vi "PXI Atten to Multiplier.vi"(8 "error in (no error)":errorcluster, 11 "Attenuation":dbl) -> (0 "error out":errorcluster, 3 "Multiplier setting":dbl[](array[numeric])=[1.0, 0.001, 1.0, 1.0, 1.0, 1.0, 1.0, 1.0])   [LabVIEW 2020]
doc: "Set multiplier values by writing the config file.\nIt also changes the multiplier global variable."
uses:
  Utility VIs/Math VIs/dB to Linear (scalar).vi
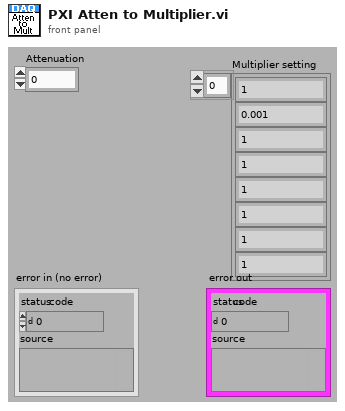
[diagram p1: front panel]
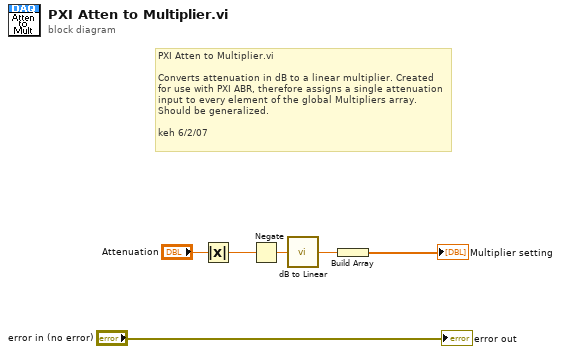
[diagram p0: block diagram]
diagram:
  # "PXI Atten to Multiplier.vi\n\nConverts attenuation in dB to a linear multiplier. Created for use with PXI ABR, therefore assigns a single attenuation input to every element of the global Multipliers array. Should be generalized.\n\nkeh 6/2/07"
  n1 = Absolute Value(x="Attenuation") -> (abs(x)=w2:dbl)
  n2 = Negate(x=w2) -> (-x=w1:dbl)
  n3 = call-poly "dB to Linear.vi"("dB"=w1) -> ("linear"=w4:dbl)
  n4 = Build Array(w4) -> (→"Multiplier setting":dbl[])
  "error out" <- "error in (no error)"
